vi "Arm Reset.vi"(11 "Reset Arm":bool) -> (1 "Done Reset":bool, 2 "Set Shoulder":dbl=-0.2, 3 "Set Elbow":dbl=-0.2)   [LabVIEW 2015]
uses:
  Sensors.vi
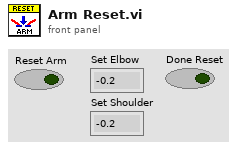
[diagram p1: front panel]
types:
  T1 = typedef "WPI_EncoderDevRef.ctl" = cluster{"DevStatus":errorcluster, "EncoderIndex":T2, "CounterIndex":T3, "DistancePerCount":dbl, "Decoding Type":T4}
  T2 = typedef "FPGA_EncoderIdx.ctl" = enum8{"Enc 0", "Enc 1", "Enc 2", "Enc 3", "Enc 4", "Enc 5", "Enc 6", "Enc 7", "Invalid"}
  T3 = typedef "FPGA_CounterCtrSystemIndex.ctl" = enum8{"Ctr 0", "Ctr 1", "Ctr 2", "Ctr 3", "Ctr 4", "Ctr 5", "Ctr 6", "Ctr 7", "Invalid"}
  T4 = typedef "WPI_EncoderType.ctl" = enum16{"1x", "2x", "4x"}
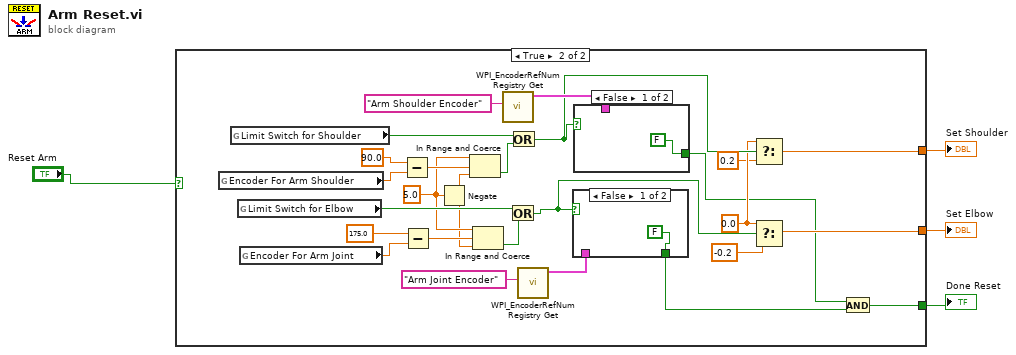
[diagram p0: block diagram]
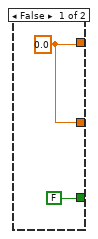
[diagram p2: hidden frame]
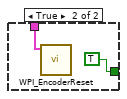
[diagram p3: hidden frame]
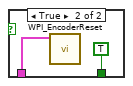
[diagram p4: hidden frame]
diagram:
  n1 = case shown="True" "Reset Arm" {
    tunnel: [w6 w14] -> w4
    tunnel: [w6 w13] -> w3
    tunnel: [FALSE w7] -> w2
    frame False {
      w6 = 0.0
    }
    frame True {
      w12 = 0.0 ("t")
      w22 = 5.0
      n2 = global read "Sensors.vi" "Encoder For Arm Shoulder"() -> (w24:dbl)
      n3 = global read "Sensors.vi" "Limit Switch for Shoulder"() -> (w20:bool)
      n4 = global read "Sensors.vi" "Limit Switch for Elbow"() -> (w27:bool)
      n5 = global read "Sensors.vi" "Encoder For Arm Joint"() -> (w30:dbl)
      n6 = Subtract(x=90.0, y=w24) -> (x-y=w25:dbl)
      n7 = Subtract(x=175.0, y=w30) -> (x-y=w28:dbl)
      n8 = Negate(x=w22) -> (-x=w21:dbl)
      n9 = In Range and Coerce(upper limit=w22, x=w25, lower limit=w21) -> (In Range?=w19:bool)  [unwired: 1 out]
      n10 = In Range and Coerce(upper limit=w22, x=w28, lower limit=w21) -> (In Range?=w26:bool)  [unwired: 1 out]
      n11 = call <vilib>:"WPI_EncoderRefNum Registry Get.vi"("refnum name"="Arm Shoulder Encoder") -> ("EncoderDevRef"=w18:T1)  [unwired: 9 in, 1 out]
      n12 = Or(x=w27, y=w26) -> (x .or. y?=w10:bool)
      n13 = Or(x=w20, y=w19) -> (x .or. y?=w16:bool)
      n14 = call <vilib>:"WPI_EncoderRefNum Registry Get.vi"("refnum name"="Arm Joint Encoder") -> ("EncoderDevRef"=w17:T1)  [unwired: 9 in, 1 out]
      n15 = case shown="False" w10 {
        tunnel: w17 -> [_ w38]
        tunnel: [FALSE TRUE] -> w8
        frame False {
        }
        frame True {
          n16 = call <vilib>:"WPI_EncoderReset.vi"("EncoderDevRef"=w38) -> ()  [unwired: 9 in, 2 out]
        }
      }
      n17 = case shown="False" w16 {
        tunnel: w18 -> [_ w35]
        tunnel: [FALSE TRUE] -> w9
        frame False {
        }
        frame True {
          n18 = call <vilib>:"WPI_EncoderReset.vi"("EncoderDevRef"=w35) -> ()  [unwired: 9 in, 2 out]
        }
      }
      n19 = Select(t=w12, s=w16, f=0.2) -> (s? t:f=w13:dbl)
      n20 = Select(t=w12, s=w10, f=-0.2) -> (s? t:f=w14:dbl)
      n21 = And(x=w9, y=w8) -> (x .and. y?=w7:bool)
    }
  }
  "Set Elbow" <- w4
  "Set Shoulder" <- w3
  "Done Reset" <- w2
